vi "Timer.vi"(7 "error in (no error)":errorcluster, 8 "Reset":bool, 9 "Pause":bool) -> (0 "error out":errorcluster, 2 "Time Has Elapsed?":bool, 3 "Elapsed Time":dbl)   [LabVIEW 2021]
doc: "This VI creates a timer program to measure the elapsed time between steps."
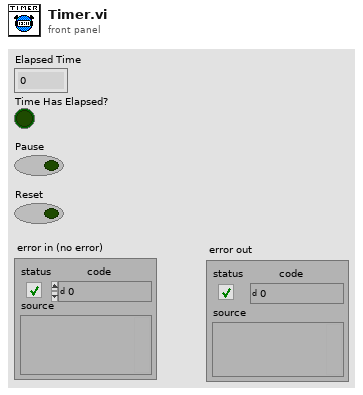
[diagram p1: front panel]
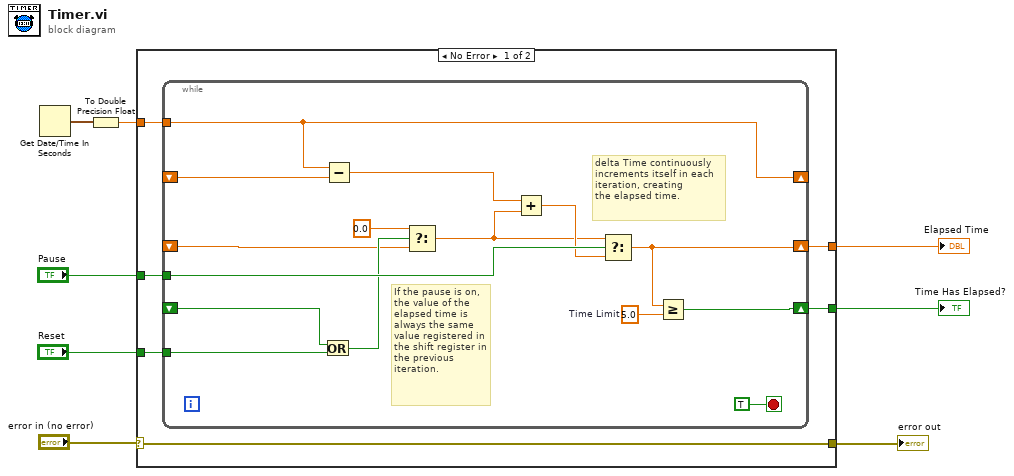
[diagram p0: block diagram]
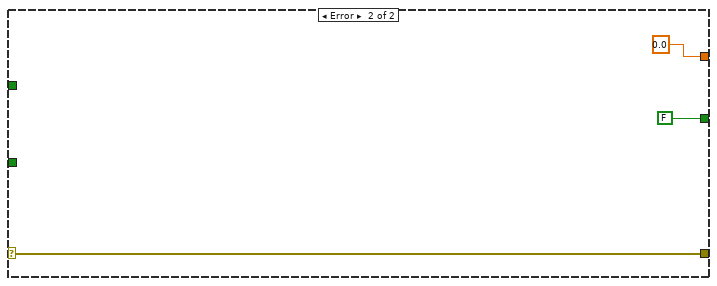
[diagram p2: hidden frame]
diagram:
  n1 = Get Date/Time In Seconds() -> (seconds since 1Jan1904=w5:timestamp)
  n2 = To Double Precision Float(number=w5) -> (double precision float=w4:dbl)
  n3 = case shown="No Error" "error in (no error)" {
    selector: "error in (no error)" -> [w10 w32]
    tunnel: [w9 0.0 ("t")] -> w8
    tunnel: [w14 FALSE] -> w7
    tunnel: "Pause" -> [w13 _]
    tunnel: w4 -> [w12 _]
    tunnel: "Reset" -> [w11 _]
    tunnel: [w10 w32] -> w1
    frame No Error {
      n4 = while {
        shift-right: [w28] -> w14
        shift-left: _ -> [w21]
        shift-right: [w24] -> _
        shift-left: _ -> [w26]
        shift-right: [w19] -> w9
        shift-left: _ -> [w16]
        tunnel: w13 -> [w25]
        tunnel: w12 -> [w24]
        tunnel: w11 -> [w20]
        stop <- TRUE stop-if-true
        w27 = 5.0  # Time Limit
        # "delta Time continuously increments itself in each iteration, creating\nthe elapsed time."
        # "If the pause is on, the value of the elapsed time is always the same value registered in the shift register in the previous iteration."
        n5 = Or(x=w21, y=w20) -> (x .or. y?=w18:bool)
        n6 = Subtract(x=w24, y=w26) -> (x-y=w23:dbl)
        n7 = Select(t=0.0, s=w18, f=w16) -> (s? t:f=w15:dbl)
        n8 = Add(x=w23, y=w15) -> (x+y=w22:dbl)
        n9 = Select(t=w15, s=w25, f=w22) -> (s? t:f=w19:dbl)
        n10 = Greater Or Equal?(x=w19, y=w27) -> (x >= y?=w28:bool)
      }
    }
    frame Error {
    }
  }
  "Elapsed Time" <- w8
  "Time Has Elapsed?" <- w7
  "error out" <- w1
